vi "Register Item(parentObject).vi"(8 "error in (no error)":errorcluster, 9 "New Object Name":string, 10 "Owner Fully Qualified Name":string, 11 "Registry in":refnum<data-value>) -> (0 "error out":errorcluster, 2 "New UniqueName Object":refnum<class "UniqueName.lvclass">, 3 "Registry":refnum<data-value>)   [LabVIEW 2014]
uses:
  NameRegistry.lvclass
  UniqueNameClass/UniqueName.lvclass
  UniquenessCriteria/UniquenessCriteria.lvclass
  UniqueNameClass/Key.ctl
  UniqueName.lvlib
  NameIncrementAlgorithm/StringIncrementAlgorithm.lvclass
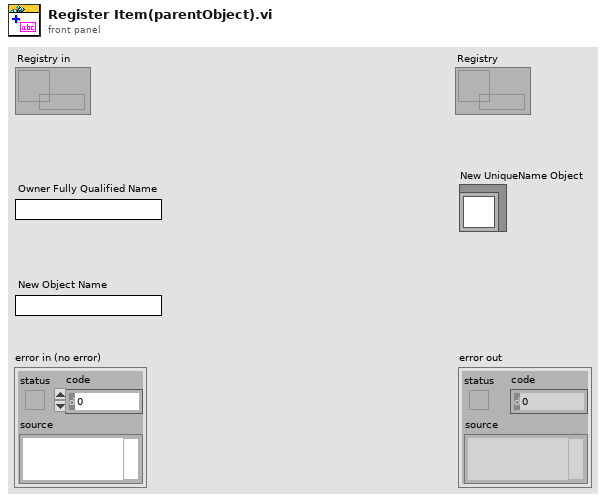
[diagram p1: front panel]
types:
  T1 = typedef "UniqueName.lvlib/Key.ctl" = enum16{"Fully Qualified Name", "Unique Name", "Given Name", "Parent Fully Qualified Name"}
  T2 = typedef "UniqueName.lvlib/UniquenessCriteria.lvclass/Criteria.ctl" = enum16{"Globally-Unique Fully Qualified Name", "Globally-Unique Name"}
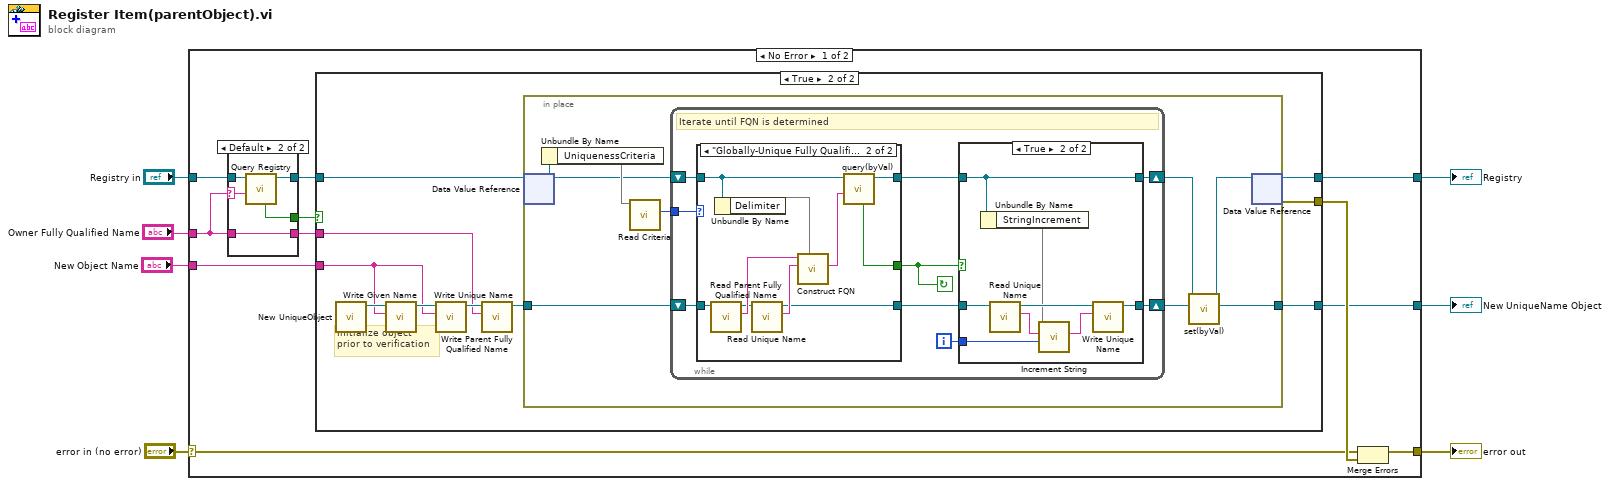
[diagram p0: block diagram]
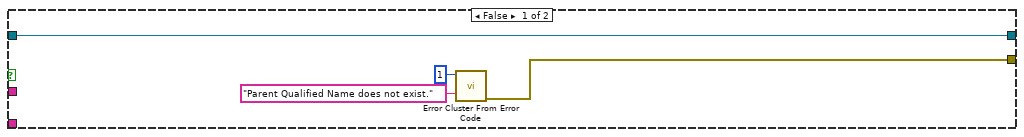
[diagram p2: hidden frame]
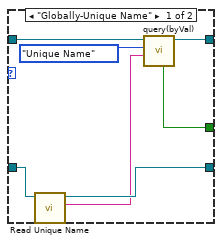
[diagram p4: hidden frame]
diagram:
  n1 = case shown="No Error" "error in (no error)" {
    selector: "error in (no error)" -> [w16 w83]
    tunnel: "Registry in" -> [w14 w84]
    tunnel: [w18 w84] -> w6
    tunnel: [w15 w83] -> w4
    tunnel: "Owner Fully Qualified Name" -> [w12 _]
    tunnel: "New Object Name" -> [w10 _]
    tunnel: [w8 _] -> w1
    frame No Error {
      n2 = case shown="Default" w12 {
        selector: w12 -> [_ w80]
        tunnel: w14 -> [w77 w82]
        tunnel: [w77 w81] -> w13
        tunnel: [_ w79] -> w11
        tunnel: [_ w78] -> w9
        tunnel: w12 -> [_ w78]
        frame "\u0000" {
        }
        frame Default {
          n3 = call "Query Registry.vi"("Search string"=w80, "Registry in"=w82) -> ("Registry"=w81:refnum<data-value>, "found?"=w79:bool)  [unwired: 5 in, 3 out]
        }
      }
      n4 = case shown="True" w11 {
        tunnel: [w22 w32] -> w18
        tunnel: [w20 w31] -> w17
        tunnel: w13 -> [w22 w25]
        tunnel: w10 -> [_ w27]
        tunnel: w9 -> [_ w26]
        tunnel: [_ w23] -> w8
        frame False {
          n5 = call <vilib>:"Error Cluster From Error Code.vi"("error message (\"\")"="Parent Qualified Name does not exist." ("error message (\"\")"), "error code (0)"=1) -> ("error out"=w20:errorcluster)  [unwired: 7 in]
        }
        frame True {
          # "Initialize object\nprior to verification"
          n6 = call "New UniqueObject.vi"() -> ("UniqueName out"=w30:refnum<class "UniqueName.lvclass">)  [unwired: 11 in]
          n7 = call "Write Given Name.vi"("Given Name"=w27, "UniqueName in"=w30) -> ("UniqueName out"=w28:refnum<class "UniqueName.lvclass">)  [unwired: 9 in]
          n8 = call "Write Unique Name.vi"("Unique Name"=w27, "UniqueName in"=w28) -> ("UniqueName out"=w29:refnum<class "UniqueName.lvclass">)  [unwired: 9 in]
          n9 = call "Write Parent Fully Qualified Name.vi"("Parent Fully Qualified Name"=w26, "UniqueName in"=w29) -> ("UniqueName out"=w24:refnum<class "UniqueName.lvclass">)  [unwired: 9 in]
          n10 = in-place {
            in-place-border: w24 -> [w38]
            in-place-border: [w35] -> w23
            n11 = in-place-dvr #1(w25) -> (w37:refnum<class "NameRegistry.lvclass">)  [unwired: 1 out]
            n12 = Unbundle By Name(w37) -> ("UniquenessCriteria"=w40)
            n13 = call "Read Criteria.vi"("UniquenessCriteria in"=w40) -> ("Criteria"=w39:T2)  [unwired: 9 in, 1 out]
            n14 = while {
              tunnel: w39 -> [w49]
              shift-right: [w47] -> w36
              shift-left: w38 -> [w46]
              shift-right: [w41] -> w34
              shift-left: w37 -> [w43]
              i -> [w44]
              stop <- w45 continue-if-true
              # "Iterate until FQN is determined"
              n15 = case shown="\"Globally-Unique Fully Qualified Name\"" w49 {
                tunnel: [w63 w70] -> w45
                tunnel: w46 -> [w66 w74]
                tunnel: [w65 w72] -> w48
                tunnel: w43 -> [w64 w68]
                tunnel: [w60 w69] -> w42
                frame "Globally-Unique Name" {
                  n16 = call "Read Unique Name.vi"("UniqueName in"=w66) -> ("Unique Name"=w61:string, "UniqueName out"=w65:refnum<class "UniqueName.lvclass">)  [unwired: 9 in]
                  n17 = call "query(byVal).vi"("Search string"=w61, "Search Key (FQN)"=Key."Unique Name" ("Key (FQN)"), "Instance"=w64) -> ("Instance"=w60:refnum<class "NameRegistry.lvclass">, "found?"=w63:bool)  [unwired: 5 in, 2 out]
                }
                frame "Globally-Unique Fully Qualified Name" {
                  n18 = call "Read Parent Fully Qualified Name.vi"("UniqueName in"=w74) -> ("Parent Fully Qualified Name"=w76:string, "UniqueName out"=w73:refnum<class "UniqueName.lvclass">)  [unwired: 9 in]
                  n19 = Unbundle By Name(w68) -> ("Delimiter"=w67)
                  n20 = call "Read Unique Name.vi"("UniqueName in"=w73) -> ("Unique Name"=w75:string, "UniqueName out"=w72:refnum<class "UniqueName.lvclass">)  [unwired: 9 in]
                  n21 = call "Construct FQN.vi"("Delimiter"=w67, "Name"=w75, "Parent FQN"=w76) -> ("FQN"=w71:string)  [unwired: 8 in]
                  n22 = call "query(byVal).vi"("Search string"=w71, "Instance"=w68) -> ("Instance"=w69:refnum<class "NameRegistry.lvclass">, "found?"=w70:bool)  [unwired: 6 in, 2 out]
                }
              }
              n23 = case shown="True" w45 {
                tunnel: w48 -> [w51 w58]
                tunnel: [w51 w59] -> w47
                tunnel: w44 -> [_ w54]
                tunnel: w42 -> [w50 w53]
                tunnel: [w50 w53] -> w41
                frame False {
                  # "Name already unique"
                }
                frame True {
                  n24 = Unbundle By Name(w53) -> ("StringIncrement"=w52)
                  n25 = call "Read Unique Name.vi"("UniqueName in"=w58) -> ("Unique Name"=w56:string, "UniqueName out"=w57:refnum<class "UniqueName.lvclass">)  [unwired: 9 in]
                  n26 = call "Increment String.vi"("Numeric"=w54, "Input String"=w56, "String Increment Algorithm"=w52) -> ("Incremented String"=w55:string)  [unwired: 8 in]
                  n27 = call "Write Unique Name.vi"("Unique Name"=w55, "UniqueName in"=w57) -> ("UniqueName out"=w59:refnum<class "UniqueName.lvclass">)  [unwired: 9 in]
                }
              }
            }
            n28 = call "set(byVal).vi"("UniqueName in"=w36, "NameRegistry in"=w34) -> ("UniqueName out"=w35:refnum<class "UniqueName.lvclass">, "NameRegistry out"=w33:refnum<class "NameRegistry.lvclass">)  [unwired: 7 in, 1 out]
            n29 = in-place-dvr #1(w33) -> (w32:refnum<data-value>, w31:errorcluster)
          }
        }
      }
      n30 = Merge Errors(w16, w17) -> (w15:errorcluster)
    }
    frame Error {
    }
  }
  "error out" <- w4
  "Registry" <- w6
  "New UniqueName Object" <- w1
